vi "InitDMA.vi"(8 "error in (no error)":errorcluster, 11 "FpgaRef5782 in":refnum<class "FpgaRef5782.lvclass">) -> (0 "error out":errorcluster, 3 "FpgaRef5782 out":refnum<class "FpgaRef5782.lvclass">)   [LabVIEW 2018, in "FpgaRef5782.lvclass"]
uses:
  FpgaRef5782.lvclass
  FpgaRef5782.lvclass/FpgaRef5782.ctl
  <vilib>/rvi/interface/common/niFpgaWaitOnOcc.vi
  <vilib>/Utility/error.llb/Error Cluster From Error Code.vi
  <vilib>/rvi/interface/nirviMethod/nirviMethod.xnode
  5782 FPGA ref.ctl
  <vilib>/rvi/errors/niLvFpgaMergeErrorWithErrorCode.vi
  <vilib>/FPGAPlugInAG/Dynamic/niLvFpga_StartFifo_Dynamic.vi
  <vilib>/FPGAPlugInAG/Dynamic/niLvFpga_ConfigureFifo_Dynamic.vi
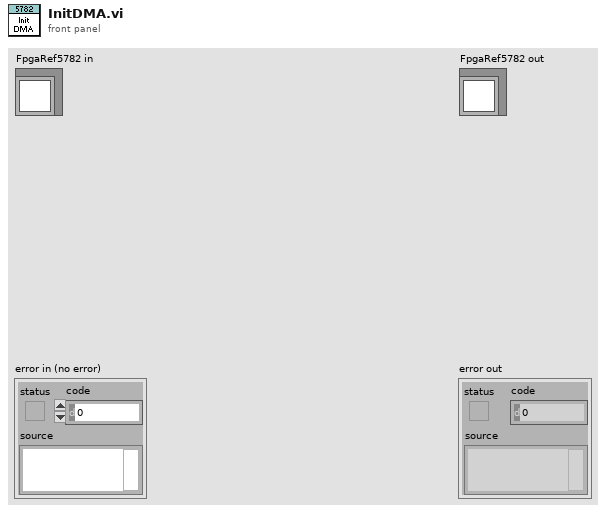
[diagram p1: front panel]
types:
  T1 = typedef "5782 FPGA ref.ctl" = refnum<k20>
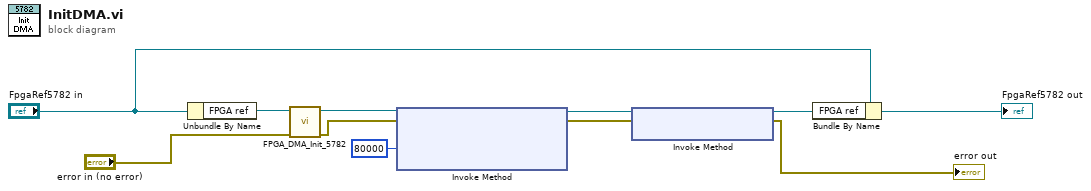
[diagram p0: block diagram]
diagram:
  n1 = Unbundle By Name("FpgaRef5782 in") -> ("FPGA ref"=w11:T1)
  n2 = call "FPGA_DMA_Init_5782.vi"("error in (no error)"="error in (no error)", "FPGA VI Reference"=w11) -> ("error out"=w2:errorcluster, "FPGA VI Out"=w5:T1)  [unwired: 7 in, 1 out]
  n3 = xnode "Invoke Method"("FPGA VI Reference In"=w5, "error in"=w2, "Requested Depth"=u32 80000 ("Depth")) -> ("FPGA VI Reference Out"=w4:T1, "error out"=w6:errorcluster)  [unwired: 1 out]
  n4 = xnode "Invoke Method"("FPGA VI Reference In"=w4, "error in"=w6) -> ("FPGA VI Reference Out"=w3:T1, "error out"=→"error out":errorcluster)
  n5 = Bundle By Name(cluster="FpgaRef5782 in", "FPGA ref"=w3) -> (→"FpgaRef5782 out":refnum<class "FpgaRef5782.lvclass">)
